vi "Check Ready to Deploy.vi"(8 "error in (no error)":errorcluster, 10 "Resource":refnum<class "DeployResource.lvclass">, 11 "DeployTarget in":refnum<class "RP2040Platform.lvclass">) -> (0 "error out":errorcluster, 2 "Ready to Deploy":bool, 3 "DeployTarget out":refnum<class "RP2040Platform.lvclass">)   [LabVIEW 2020, in "RP2040.lvlib" / "RP2040Platform.lvclass"]
uses:
  RP2040Platform.lvclass
  VisaResource/VisaResource.lvclass
  4ea13893-8da5-4792-9cbf-2551c97df416.vi
  <vilib>/Instr/_visa.llb/VISA Configure Serial Port (Instr).vi
  Builds/picoG/ppl/PicoG-Core.lvlibp/PicoG-Processor/PicoG-Core/DeployResource/DeployResource.lvclass
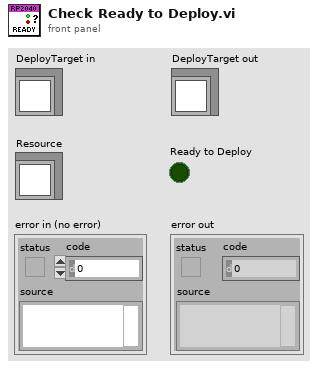
[diagram p1: front panel]
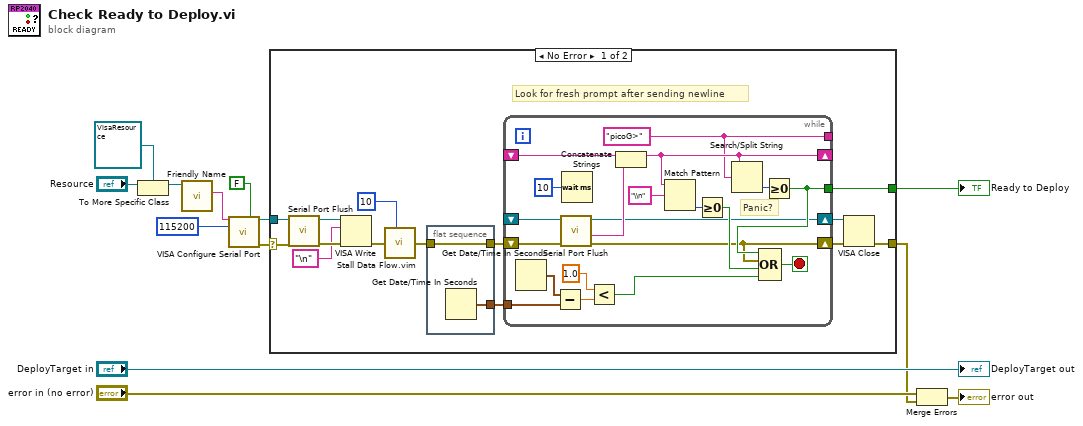
[diagram p0: block diagram]
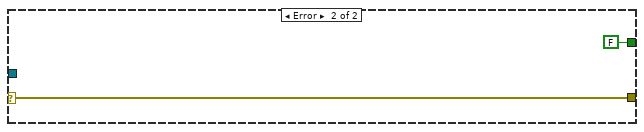
[diagram p2: hidden frame]
diagram:
  n1 = To More Specific Class(target class=refnum<class "VisaResource.lvclass"> refnum ("RP2040:VisaResource"), reference="Resource") -> (specific class reference=w9:refnum<class "VisaResource.lvclass">)  [unwired: 1 in, 1 out]
  n2 = call-dynamic "Friendly Name.vi"("VisaResource in"=w9) -> ("Friendly Name"=w8:string)  [unwired: 8 in, 2 out]
  n3 = call-poly "VISA Configure Serial Port"("VISA resource name"=w8, "Enable Termination\nChar (T)"=FALSE ("Enable Termination\nChar (T)"), "baud rate (9600)"=u32 115200) -> ("VISA resource name out"=w5:refnum<visa-resource-name>, "error out"=w4:errorcluster)  [unwired: 11 in]
  n4 = case shown="No Error" w4 {
    selector: w4 -> [w26 w50]
    tunnel: w5 -> [w27 _]
    tunnel: [w17 FALSE] -> w3
    tunnel: [w14 w50] -> w1
    frame No Error {
      # "Look for fresh prompt after sending newline"
      n5 = call "Serial Port Flush.vi"("error in (no error)"=w26, "VISA resource name"=w27) -> ("error out"=w25:errorcluster, "duplicate VISA resource name"=w24:refnum<visa-resource-name>)  [unwired: 7 in, 1 out]
      n6 = VISA Write(VISA resource name=w24, write buffer="\n" ("string"), error in (no error)=w25) -> (error out=w20:errorcluster)  [unwired: 2 out]
      n7 = call "Stall Data Flow.vim"("value in"=w20, "milliseconds to wait"=u32 10) -> ("value out"=w19:errorcluster)  [unwired: 1 out]
      n8 = flat-sequence {
        tunnel: w19 -> [w29]
        tunnel: [w29] -> w21
        tunnel: [w28] -> w22
        frame #0 {
          n9 = Get Date/Time In Seconds() -> (seconds since 1Jan1904=w28:timestamp)
        }
      }
      n10 = while {
        shift-right: [w30] -> w15
        shift-left: w21 -> [w33]
        shift-right: [w31] -> w16
        shift-left: _ -> [w34]
        tunnel: w22 -> [w49]
        shift-right: [w38] -> _
        shift-left: _ -> [w42]
        tunnel: [w36] -> _
        tunnel: [w35] -> w17
        stop <- w45 stop-if-true
        w36 = "picoG>" ("regular expression")
        # "Panic?"
        n11 = Get Date/Time In Seconds() -> (seconds since 1Jan1904=w48:timestamp)
        n12 = Subtract(x=w48, y=w49) -> (x-y=w47:dbl)
        n13 = call "Serial Port Flush.vi"("error in (no error)"=w33, "VISA resource name"=w34) -> ("error out"=w30:errorcluster, "FLUSHED CHARS"=w32:string, "duplicate VISA resource name"=w31:refnum<visa-resource-name>)  [unwired: 7 in]
        n14 = Wait (ms)(milliseconds to wait=u32 10) -> ()  [unwired: 1 out]
        n15 = Less?(x=1.0, y=w47) -> (x < y?=w44:bool)
        n16 = Concatenate Strings(w42, w32) -> (w38:string)
        n17 = Match Pattern(string=w38, regular expression="\\n") -> (offset past match=w40:i32)  [unwired: 1 in, 3 out]
        n18 = Greater Or Equal To 0?(x=w40) -> (x >= 0?=w39:bool)
        n19 = Search/Split String(string=w38, search string/char (-)=w36) -> (offset of match=w37:i32)  [unwired: 1 in, 2 out]
        n20 = Greater Or Equal To 0?(x=w37) -> (x >= 0?=w35:bool)
        n21 = Compound Arithmetic op=OR(w35, w30, w39, w44) -> (w45:bool)
      }
      n22 = VISA Close(VISA resource name=w16, error in (no error)=w15) -> (error out=w14:errorcluster)
    }
    frame Error {
    }
  }
  "Ready to Deploy" <- w3
  n23 = Merge Errors("error in (no error)", w1) -> (→"error out":errorcluster)
  "DeployTarget out" <- "DeployTarget in"
